vi "Update GPU Graph.vi"(6 "f0":dbl, 8 "error in (no error)":errorcluster, 9 "df":dbl, 10 "Plot":sgl[](array[numeric]), 11 "Application Manager in":refnum<class "Application Manager.lvclass">) -> (0 "error out":errorcluster, 3 "Application Manager out":refnum<class "Application Manager.lvclass">)   [LabVIEW 2020, in "Application Manager.lvlib" / "Application Manager.lvclass"]
uses:
  Application Manager.lvclass
  <vilib>/ActorFramework/Message Enqueuer/Message Priority.ctl
  Application Manager.lvclass/Application Manager.ctl
  Simple UI/Simple UI Messages/Update GPU Graph Msg/Update GPU Graph Msg.lvclass/Update GPU Graph Msg.ctl
  <vilib>/ActorFramework/Message Enqueuer/Message Enqueuer.lvclass/Message Enqueuer.ctl
  <vilib>/ActorFramework/Message Enqueuer/Enqueue.vi
  Simple UI/Simple UI Messages/Update GPU Graph Msg/Update GPU Graph Msg.lvclass
  C:/Program Files/National Instruments/LabVIEW 2026/vi.lib/ActorFramework/Message/Message.lvclass
  <vilib>/ActorFramework/Message Priority Queue/Priority Enqueue.vi
  <vilib>/ActorFramework/Message Enqueuer/Message Enqueuer.lvclass
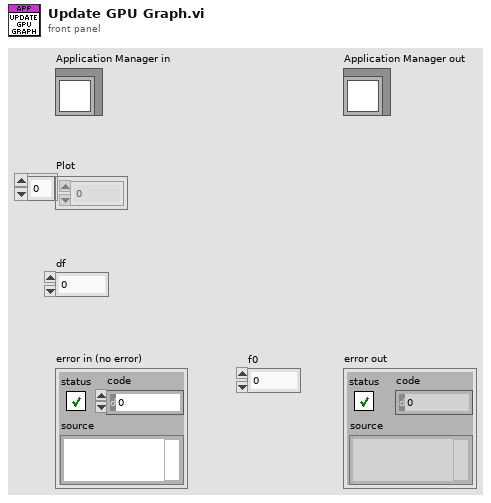
[diagram p1: front panel]
types:
  T1 = typedef "Actor Framework.lvlib/Message Enqueuer.lvclass/Message Priority.ctl" = enum16{"Low", "Normal", "High"}
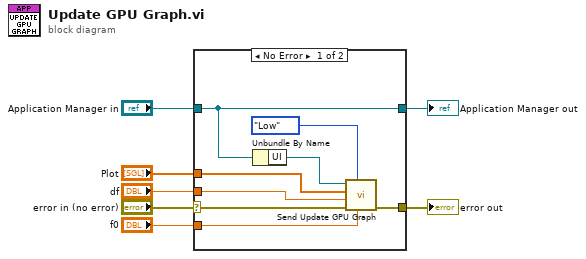
[diagram p0: block diagram]
diagram:
  n1 = case shown="No Error" "error in (no error)" {
    selector: "error in (no error)" -> [w15 w17]
    tunnel: [w14 w17] -> w6
    tunnel: [w11 w16] -> w4
    tunnel: "Application Manager in" -> [w11 w16]
    tunnel: "df" -> [w13 _]
    tunnel: "Plot" -> [w12 _]
    tunnel: "f0" -> [w8 _]
    frame No Error {
      n2 = Unbundle By Name(w11) -> ("UI"=w10:refnum<class "Message Enqueuer.lvclass">)
      n3 = call "Send Update GPU Graph.vi"("f0"=w8, "Message Priority (Normal)"=Message_Priority."Low", "error in (no error)"=w15, "df"=w13, "Plot"=w12, "Message Enqueuer"=w10) -> ("error out"=w14:errorcluster)  [unwired: 4 in, 1 out]
    }
    frame Error {
    }
  }
  "error out" <- w6
  "Application Manager out" <- w4
